vi "Send Message over UDP.vi"(0 "message":T1, 1 "UDP receiver port":u16, 5 "UDP connection ID":refnum<k16>, 9 "timeout (25000 ms)":i32=25200, 11 "error in":errorcluster) -> (6 "message string":string, 10 "timed out?":bool, 15 "error out":errorcluster)   [LabVIEW 2009, in "AMC.lvlib"]
doc: "Sends a message to a receiver process over UDP.\n\nIf <b>UDP connection ID</b> is wired, the message will be sent using that connection.\n\nIf <b>UDP connection ID</b> is unwired, the message will be sent using the same connection as <b>UDP Dispatcher.vi</b>."
uses:
  AMC.lvlib
  Message.ctl
  <vilib>/NI/Tools/Keyed Array/KeyedArray.ctl
  <vilib>/NI/Tools/Keyed Array/Tools_KeyedArray.lvlib
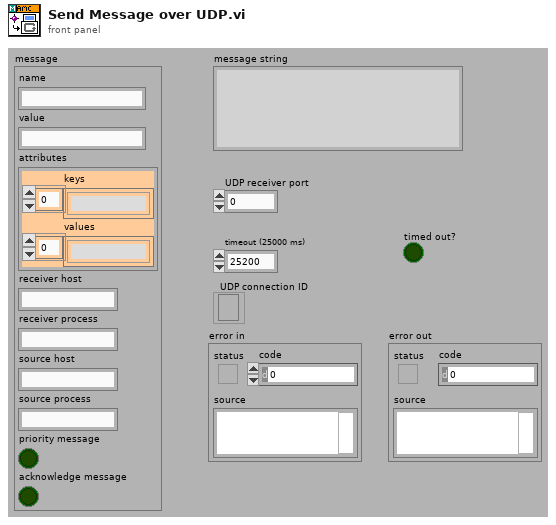
[diagram p1: front panel]
types:
  T1 = typedef "AMC.lvlib/Message.ctl" = cluster{"name":string, "value":string, "attributes":T2, "receiver host":string, "receiver process":string, "source host":string, "source process":string, "priority message":bool, "acknowledge message":bool}
  T2 = typedef "Tools_KeyedArray.lvlib/KeyedArray.ctl" = cluster{"keys":string[], "values":string[]}
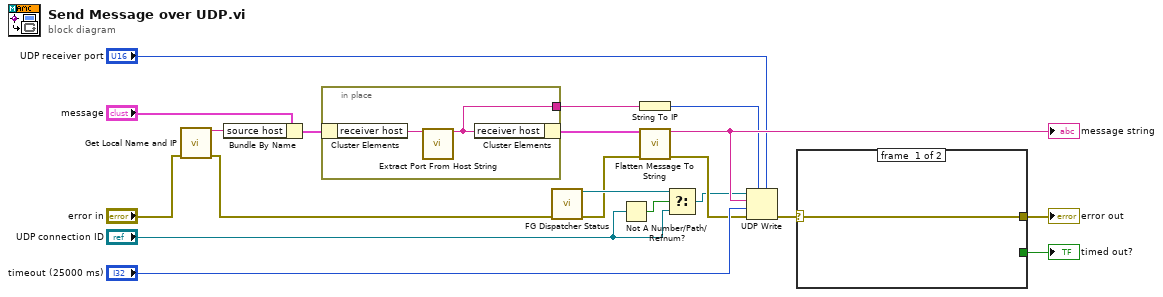
[diagram p0: block diagram]
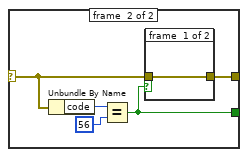
[diagram p2: hidden frame]
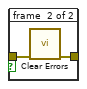
[diagram p3: hidden frame]
diagram:
  n1 = call "Get Local Name and IP.vi"("error in"="error in") -> ("name"=w5:string, "error out"=w4:errorcluster)  [unwired: 11 in, 2 out]
  n2 = Bundle By Name(cluster="message", "source host"=w5) -> (w3:T1)
  n3 = in-place {
    in-place-border: [w21] -> w1
    n4 = in-place-cluster #1(w3) -> ("receiver host"=w22:string)
    n5 = call "Extract Port From Host String.vi"("host in"=w22) -> ("host out"=w21:string)  [unwired: 12 in, 2 out]
    n6 = in-place-cluster #1("receiver host"=w21) -> (w2:T1)
  }
  n7 = call "FG Dispatcher Status.vi"("error in"=w4) -> ("UDP connection ID"=w8:refnum<k16>, "error out"=w6:errorcluster)  [unwired: 12 in, 1 out]
  n8 = Not A Number/Path/Refnum?(number/path/refnum="UDP connection ID") -> (NaN/Path/Refnum?=w9:bool)
  n9 = String To IP(1:w1) -> (0:w12:u32)
  n10 = call "Flatten Message To String.vi"("message"=w2, "error in"=w6) -> ("message string"=w17:string, "error out"=w10:errorcluster)  [unwired: 12 in]
  "message string" <- w17
  n11 = Select(t=w8, s=w9, f="UDP connection ID") -> (s? t:f=w7:refnum<k16>)
  n12 = UDP Write(address=w12, port or service name="UDP receiver port", connection ID=w7, data in=w17, 8:w10, 9:"timeout (25000 ms)") -> (error out=w11:errorcluster)  [unwired: 1 out]
  n13 = case shown="Error" w11 {
    selector: w11 -> [w23 w26]
    tunnel: [w23 w25] -> w20
    tunnel: [_ w24] -> w15
    frame #0 {
    }
    frame #1 {
      n14 = Unbundle By Name(w26) -> ("code"=w28:i32)
      n15 = Equal?(x=w28, y=56) -> (x = y?=w24:bool)
      n16 = case shown="True" w24 {
        tunnel: w26 -> [w29 w31]
        tunnel: [w29 w30] -> w25
        frame #0 {
        }
        frame #1 {
          n17 = call <vilib>:"Clear Errors.vi"("error in (no error)"=w31) -> ("error out"=w30:errorcluster)  [unwired: 6 in]
        }
      }
    }
  }
  "error out" <- w20
  "timed out?" <- w15
